vi "Start Helper Loop.vi"(8 "error in (no error)":errorcluster, 11 "DELAY Timeout":i32) -> (0 "error out":errorcluster)   [LabVIEW 2020, in "Acquisition.lvlib"]
doc: "Starts the Helper Loop fo continuous tasks\n_____\nCreated using Delacor QMH Event Scripter 5.0.0.112."
uses:
  Acquisition.lvlib
  Start Helper Loop Argument--cluster.ctl
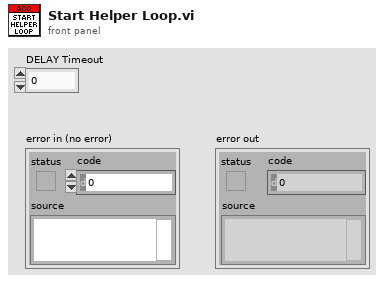
[diagram p1: front panel]
types:
  T1 = typedef "Acquisition.lvlib/Start Helper Loop Argument--cluster.ctl" = cluster{"DELAY Timeout":i32}
  T2 = typedef "Acquisition.lvlib/Request Events--cluster.ctl" = cluster{"Stop Module":refnum<user-event>, "Show Panel":refnum<user-event>, "Hide Panel":refnum<user-event>, "Get Module Execution Status":refnum<user-event>, "Show Diagram":refnum<user-event>, "Start Helper Loop":refnum<user-event>, "Stop Helper Loop":refnum<user-event>, "ACQ Config":refnum<user-event>}
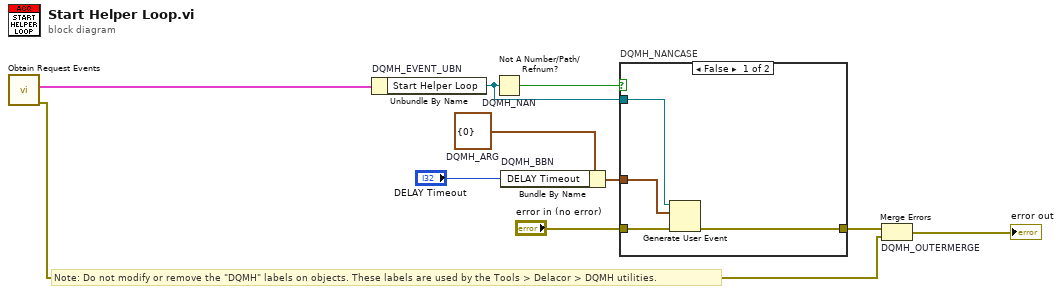
[diagram p0: block diagram]
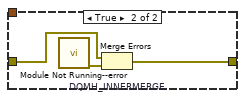
[diagram p2: hidden frame]
diagram:
  w4 = T1 {"DELAY Timeout"=0}  # DQMH_ARG
  # "Note: Do not modify or remove the \"DQMH\" labels on objects. These labels are used by the Tools > Delacor > DQMH utilities."
  n1 = call "Obtain Request Events.vi"() -> ("error out"=w3:errorcluster, "Acquisition Request Events"=w2:T2)  [unwired: 10 in]
  n2 = Unbundle By Name "DQMH_EVENT_UBN"(w2) -> ("Start Helper Loop"=w6:refnum<user-event>)
  n3 = Not A Number/Path/Refnum? "DQMH_NAN"(number/path/refnum=w6) -> (NaN/Path/Refnum?=w7:bool)
  n4 = Bundle By Name "DQMH_BBN"(cluster=w4, "DELAY Timeout"="DELAY Timeout") -> (w8:T1)
  n5 = case "DQMH_NANCASE" shown="False" w7 {
    tunnel: "error in (no error)" -> [w14 w17]
    tunnel: [w13 w16] -> w5
    tunnel: w6 -> [w12 _]
    tunnel: w8 -> [w11 _]
    frame False {
      n6 = Generate User Event(user event=w12, event data cluster=w11, error in=w14) -> (error out=w13:errorcluster)  [unwired: 1 in, 1 out]
    }
    frame True {
      n7 = call "Module Not Running--error.vi"() -> ("error out"=w15:errorcluster)  [unwired: 11 in]
      n8 = Merge Errors "DQMH_INNERMERGE"(w17, w15) -> (w16:errorcluster)
    }
  }
  n9 = Merge Errors "DQMH_OUTERMERGE"(w5, w3) -> (→"error out":errorcluster)
